vi "get_uncorrected_coordinates.vi"(8 "error in (no error)":errorcluster, 11 "TrajectoryCN090716SpiralScan in":refnum<class "TrajectoryCN090716SpiralScan.lvclass">) -> (0 "error out":errorcluster, 1 "y":dbl[unit][](array[numeric]), 2 "z":dbl[unit][](array[numeric]), 3 "TrajectoryCN090716SpiralScan out":refnum<class "TrajectoryCN090716SpiralScan.lvclass">, 4 "x":dbl[unit][](array[numeric]))   [LabVIEW 2010, in "TrajectoryCN090716SpiralScan.lvclass"]
uses:
  TrajectoryCN090716SpiralScan.lvclass
  common/enumerations/x_y_z_enumeration.ctl
  common/enumerations/functional_global_action_enum.ctl
  TrajectoryCN090716SpiralScan.lvclass/TrajectoryCN090716SpiralScan.ctl
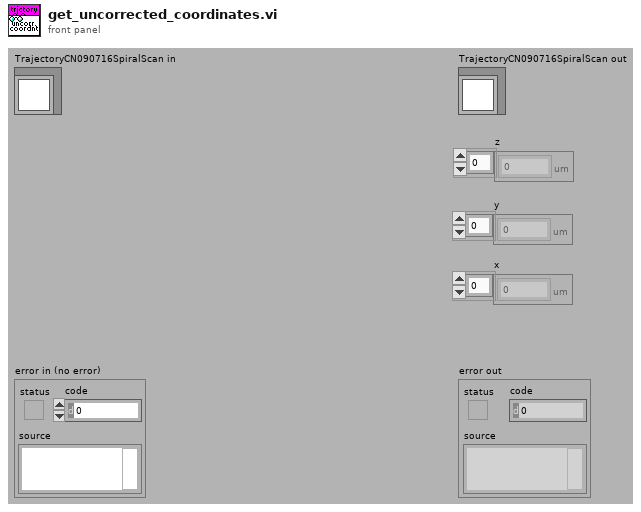
[diagram p1: front panel]
types:
  T1 = typedef "x_y_z_enumeration.ctl" = enum16{"x", "y", "z"}
  T2 = typedef "functional_global_action_enum.ctl" = enum16{"get", "set", "reset"}
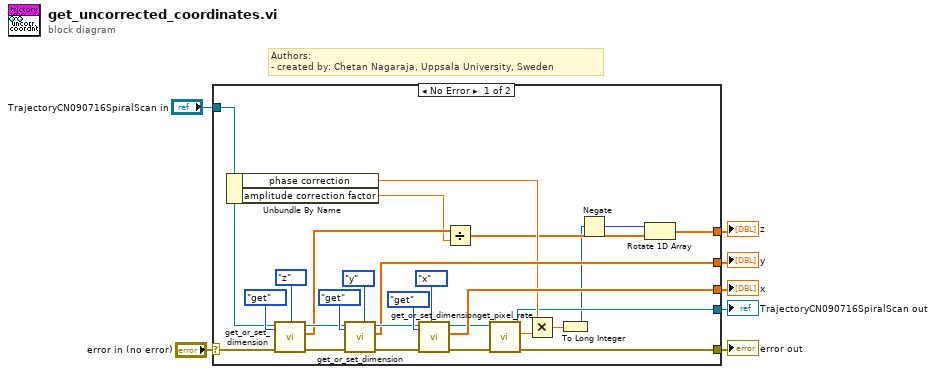
[diagram p0: block diagram]
diagram:
  # "Authors: \n- created by: Chetan Nagaraja, Uppsala University, Sweden"
  n1 = case shown="No Error" "error in (no error)" {
    selector: "error in (no error)" -> [w24 w36]
    tunnel: [w9 w36] -> w6
    tunnel: [w12 w35] -> w4
    tunnel: "TrajectoryCN090716SpiralScan in" -> [w13 w35]
    tunnel: [w23 _] -> w1
    tunnel: [w22 _] -> w2
    tunnel: [w10 _] -> w3
    frame No Error {
      n2 = Unbundle By Name(w13) -> ("phase correction"=w18:dbl[unit], "amplitude correction factor"=w20:dbl)
      n3 = call-dynamic "get_or_set_dimension.vi"("dimension"=x_y_z_enumeration."z", "action"=functional_global_action_enum."get", "error in (no error)"=w24, "GenericTrajectory in"=w13) -> ("error out"=w25:errorcluster, "pixel values out (single dimension)"=w21:dbl[unit][], "GenericTrajectory out"=w28:refnum<class "TrajectoryCN090716SpiralScan.lvclass">)  [unwired: 5 in]
      n4 = call-dynamic "get_or_set_dimension.vi"("dimension"=x_y_z_enumeration."y", "action"=functional_global_action_enum."get", "error in (no error)"=w25, "GenericTrajectory in"=w28) -> ("error out"=w27:errorcluster, "pixel values out (single dimension)"=w22:dbl[unit][], "GenericTrajectory out"=w26:refnum<class "TrajectoryCN090716SpiralScan.lvclass">)  [unwired: 5 in]
      n5 = call-dynamic "get_or_set_dimension.vi"("dimension"=x_y_z_enumeration."x", "action"=functional_global_action_enum."get", "error in (no error)"=w27, "GenericTrajectory in"=w26) -> ("error out"=w19:errorcluster, "pixel values out (single dimension)"=w23:dbl[unit][], "GenericTrajectory out"=w14:refnum<class "TrajectoryCN090716SpiralScan.lvclass">)  [unwired: 5 in]
      n6 = Divide(x=w21, y=w20) -> (x/y=w16:dbl[unit][])
      n7 = call-dynamic "get_pixel_rate.vi"("error in (no error)"=w19, "GenericTrajectory in"=w14) -> ("error out"=w9:errorcluster, "pixel rate"=w17:dbl[unit], "GenericTrajectory out"=w12:refnum<class "TrajectoryCN090716SpiralScan.lvclass">)  [unwired: 6 in, 1 out]
      n8 = Multiply(x=w18, y=w17) -> (x*y=w15:dbl)
      n9 = To Long Integer(number=w15) -> (32bit integer=w11:i32)
      n10 = Negate(x=w11) -> (-x=w8:i32)
      n11 = Rotate 1D Array(1:w16, 2:w8) -> (0:w10:dbl[unit][])
    }
    frame Error {
    }
  }
  "error out" <- w6
  "TrajectoryCN090716SpiralScan out" <- w4
  "z" <- w3
  "y" <- w2
  "x" <- w1
